vi "Analyze.vi"(0 "Analyze Distanz in":refnum<class "Analyze Distanz.lvclass">, 1 "Create Overlay?":bool, 5 "Image in":T1, 7 "Parameters":variant, 9 "Results in":variant, 11 "error in (no error)":errorcluster) -> (4 "Analyze Distanz out":refnum<class "Analyze Distanz.lvclass">, 6 "Image out":T1, 8 "Parameters out":variant, 10 "Results":variant, 15 "error out":errorcluster)   [LabVIEW 2014, in "Analyze.lvlib" / "Analyze Distanz.lvclass"]
uses:
  Analyze Distanz.lvclass
  <vilib>/vision/Image Controls.llb/IMAQ Image.ctl
  Analyze BaseClass/Analyze BaseClass.lvclass
  Utility/POLARIS Vision utility.lvlib
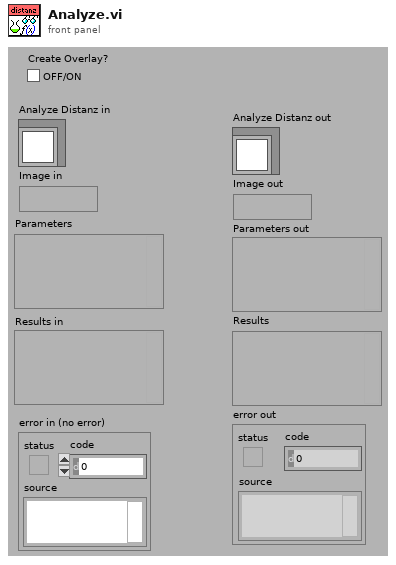
[diagram p1: front panel]
types:
  T1 = typedef "IMAQ Image.ctl" = refnum<image>
  T2 = typedef "ROI Descriptor" = cluster{"Global Rectangle":i32[], "Contours":cluster{"ID":enum32{"External", "Internal"}, "Type":u32, "Coordinates":i32[]}[]}
  T3 = cluster{"ID":enum32{"External", "Internal"}, "Type":u32, "Coordinates":i32[]}[]
  T4 = cluster{"Desired Font (Application)":enum16{"User-specified Font", "Application Font", "System Font", "Dialog Font"}, "[User-specified Font]":cluster{"Font Name":string, "Size":i16, "Strikeout?":bool, "Italic?":bool, "Underline?":bool, "Outline?":bool, "Shadow?":bool, "Bold?":bool, "Rotation Angle":dbl}, "Horizontal Alignment":i16, "Vertical Alignment":i16}
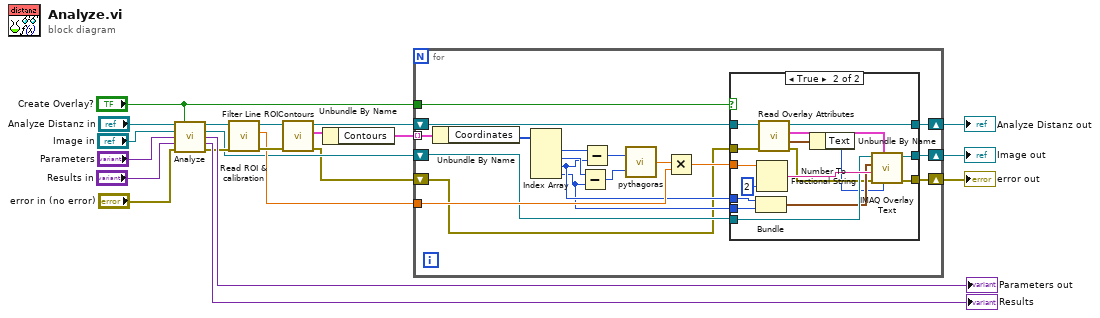
[diagram p0: block diagram]
diagram:
  n1 = call-parent "Analyze.vi"("Analyze BaseClass in"="Analyze Distanz in", "Create Overlay?"="Create Overlay?", "Image in"="Image in", "Parameters"="Parameters", "Results in"="Results in", "error in (no error)"="error in (no error)") -> ("Analyze BaseClass out"=w14:refnum<class "Analyze Distanz.lvclass">, "Image out"=w4:T1, "Parameters out"=→"Parameters out":variant, "Results"=→"Results":variant, "error out"=w13:errorcluster)  [unwired: 5 in]
  n2 = call-dynamic "Read ROI & calibration.vi"("error in (no error)"=w13, "Analyze BaseClass in"=w14) -> ("error out"=w12:errorcluster, "calibration mm/px"=w8:dbl, "Analyze BaseClass out"=w11:refnum<class "Analyze Distanz.lvclass">)  [unwired: 6 in, 1 out]
  n3 = call-dynamic "Filter Line ROIContours.vi"("error in (no error)"=w12, "Analyze BaseClass in"=w11) -> ("error out"=w3:errorcluster, "Line contours"=w10:T2, "Analyze BaseClass out"=w6:refnum<class "Analyze Distanz.lvclass">)  [unwired: 7 in]
  n4 = Unbundle By Name(w10) -> ("Contours"=w9:T3)
  n5 = for {
    tunnel: w9 -> [w39] mode=indexing
    tunnel: w8 -> [w32]
    tunnel: "Create Overlay?" -> [w31]
    shift-right: [w28] -> w5
    shift-left: w6 -> [w29]
    shift-right: [w24] -> w1
    shift-left: w4 -> [w27]
    shift-right: [w23] -> w2
    shift-left: w3 -> [w22]
    n6 = Unbundle By Name(w39) -> ("Coordinates"=w38:i32[])
    n7 = Index Array(array=w38) -> (element #1=w36:i32, element #2=w35:i32, element #3=w26:i32, element #4=w25:i32)  [unwired: 4 in]
    n8 = Subtract(x=w35, y=w25) -> (x-y=w34:i32)
    n9 = Subtract(x=w36, y=w26) -> (x-y=w37:i32)
    n10 = call "pythagoras.vi"("b"=w34, "a"=w37) -> ("c"=w33:dbl)
    n11 = Multiply(x=w33, y=w32) -> (x*y=w30:dbl)
    n12 = case shown="True" w31 {
      tunnel: w30 -> [_ w55]
      tunnel: w29 -> [w42 w58]
      tunnel: [w42 w57] -> w28
      tunnel: w27 -> [w41 w54]
      tunnel: w26 -> [_ w51]
      tunnel: w25 -> [_ w50]
      tunnel: [w41 w48] -> w24
      tunnel: [w40 w46] -> w23
      tunnel: w22 -> [w40 w45]
      frame False {
      }
      frame True {
        n13 = Bundle(w51, w50) -> (w49:cluster{i32, i32})  [unwired: 1 in]
        n14 = Number To Fractional String(number=w55, precision (6)=i16 2) -> (F-format string=w56:string)  [unwired: 2 in]
        n15 = call-dynamic "Read Overlay Attributes.vi"("error in (no error)"=w45, "Analyze BaseClass in"=w58) -> ("error out"=w47:errorcluster, "Overlay colors"=w44:cluster{"Border":u32, "Text":u32}, "Font, Size & Style"=w52:T4, "Analyze BaseClass out"=w57:refnum<class "Analyze Distanz.lvclass">)  [unwired: 5 in, 1 out]
        n16 = Unbundle By Name(w44) -> ("Text"=w43:u32)
        n17 = call "IMAQ Overlay Text"("Text Color (black)"=w43, "Font, Size & Style"=w52, "error in (no error)"=w47, "String"=w56, "Origin"=w49, "Image"=w54) -> ("error out"=w46:errorcluster, "Image Out"=w48:T1)  [unwired: 4 in]
      }
    }
  }
  "error out" <- w2
  "Analyze Distanz out" <- w5
  "Image out" <- w1
